vi "close image source.vi"(8 "error in (no error)":errorcluster, 11 "image source data":T4) -> (0 "error out":errorcluster)   [LabVIEW 2021]
uses:
  <vilib>/userDefined/High Color/IMAQdx.ctl
  <vilib>/vision/Avi1.llb/AviRefnum.ctl
  <vilib>/vision/Image Controls.llb/IMAQ Image.ctl
  <vilib>/vision/driver/NI_Vision_Acquisition_Software.lvlib
  Image-Stack-Compressor/Stack Reader Wrapper/labview vis/StackReaderWrapper.lvlib
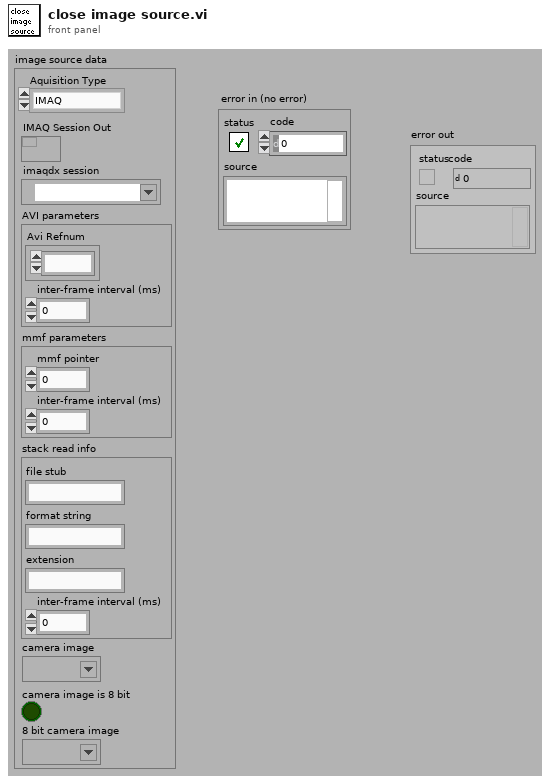
[diagram p1: front panel]
types:
  T1 = typedef "IMAQdx.ctl" = refnum<k21>
  T2 = typedef "AviRefnum.ctl" = refnum<k1>
  T3 = typedef "IMAQ Image.ctl" = refnum<image>
  T4 = cluster{"Aquisition Type":enum16{"IMAQ", "IMAQdx", "AVI", "MMF", "STACK"}, "IMAQ Session Out":refnum<k11>, "imaqdx session":T1, "AVI parameters":cluster{"Avi Refnum ":T2, "inter-frame interval (ms)":dbl}, "mmf parameters":cluster{"mmf pointer":u32, "inter-frame interval (ms)":dbl}, "stack read info":cluster{"file stub":string, "format string":string, "extension":string, "inter-frame interval (ms)":dbl}, "camera image":T3, "camera image is 8 bit":bool, "8 bit camera image":T3}
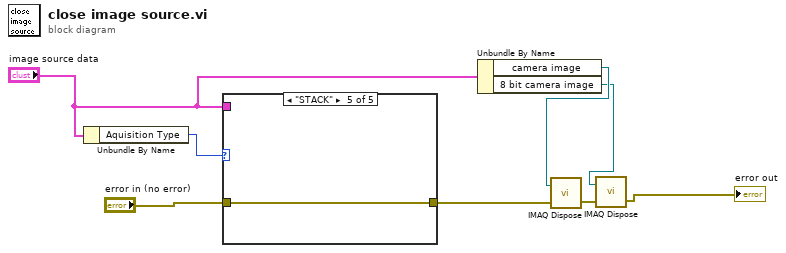
[diagram p0: block diagram]
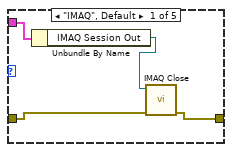
[diagram p2: hidden frame]
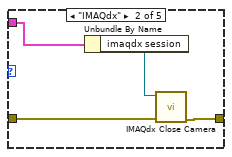
[diagram p3: hidden frame]
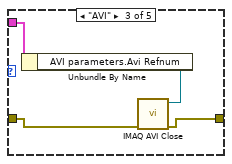
[diagram p4: hidden frame]
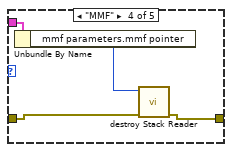
[diagram p5: hidden frame]
diagram:
  n1 = Unbundle By Name("image source data") -> ("Aquisition Type"=w7:enum16{"IMAQ", "IMAQdx", "AVI", "MMF", "STACK"})
  n2 = case shown="\"STACK\"" w7 {
    tunnel: "image source data" -> [w12 w16 w18 w22 _]
    tunnel: "error in (no error)" -> [w10 w14 w20 w24 w25]
    tunnel: [w9 w13 w19 w23 w25] -> w5
    frame "IMAQ", Default {
      n3 = Unbundle By Name(w12) -> ("IMAQ Session Out"=w11:refnum<k11>)
      n4 = call <vilib>:"IMAQ Close.vi"("error in (no error)"=w10, "IMAQ Session In"=w11) -> ("error out"=w9:errorcluster)  [unwired: 9 in]
    }
    frame "IMAQdx" {
      n5 = Unbundle By Name(w16) -> ("imaqdx session"=w15:T1)
      n6 = call <vilib>:"IMAQdx Close Camera.vi"("error in"=w14, "Session In"=w15) -> ("error out"=w13:errorcluster)  [unwired: 9 in]
    }
    frame "AVI" {
      n7 = Unbundle By Name(w18) -> ("AVI parameters.Avi Refnum"=w17:T2)
      n8 = call "IMAQ AVI Close"("error in (no error)"=w20, "Avi Refnum"=w17) -> ("error out"=w19:errorcluster)  [unwired: 9 in]
    }
    frame "MMF" {
      n9 = Unbundle By Name(w22) -> ("mmf parameters.mmf pointer"=w21:u32)
      n10 = call "destroy Stack Reader.vi"("error in (no error)"=w24, "sr"=w21) -> ("error out"=w23:errorcluster)  [unwired: 8 in, 1 out]
    }
    frame "STACK" {
    }
  }
  n11 = Unbundle By Name("image source data") -> ("camera image"=w2:T3, "8 bit camera image"=w1:T3)
  n12 = call "IMAQ Dispose"("Image"=w2, "error in (no error)"=w5) -> ("error out"=w4:errorcluster)  [unwired: 4 in]
  n13 = call "IMAQ Dispose"("Image"=w1, "error in (no error)"=w4) -> ("error out"=→"error out":errorcluster)  [unwired: 4 in]
